vi "MoveChanGroup.vi"(7 "Up (T) / Down (F)":bool, 8 "error in (no error)":errorcluster, 9 "Rate Class":T1, 10 "ChanGroup":i32, 11 "Chassis Cfg":refnum<class "ChassisCfg.lvclass">) -> (0 "error out":errorcluster, 1 "Disregard":bool, 2 "ChanGroup Out":i32, 3 "Chassis Cfg":refnum<class "ChassisCfg.lvclass">)   [LabVIEW 2012, in "Configuration Grandmaster.lvlib" / "ChassisCfg.lvclass"]
uses:
  ChassisCfg.lvclass
  Common/Controls/TE_Designator.ctl
  ChassisCfg.lvclass/ChassisCfg.ctl
  Class Timing Group/TimingGrp.lvclass
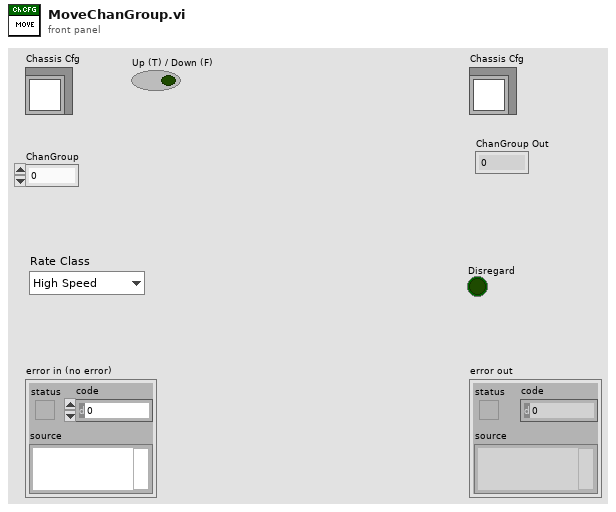
[diagram p1: front panel]
types:
  T1 = typedef "TE_Designator.ctl" = enum16{"High Speed", "Low Speed"}
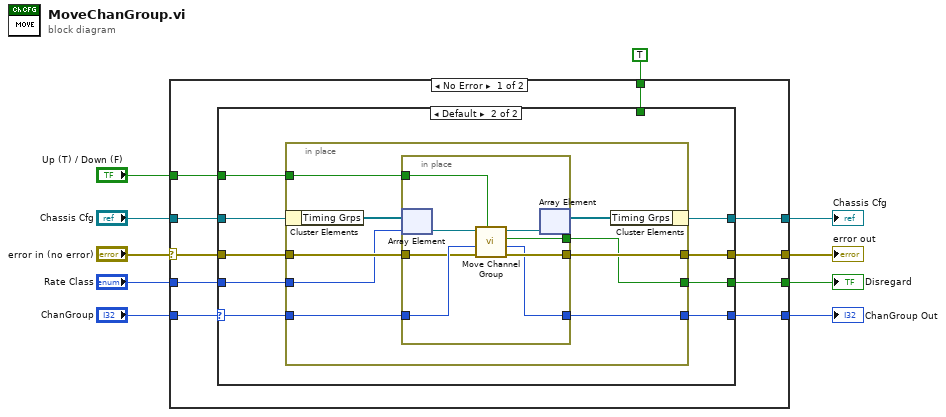
[diagram p0: block diagram]
diagram:
  n1 = case shown="No Error" "error in (no error)" {
    selector: "error in (no error)" -> [w19 w54]
    tunnel: [w17 w54] -> w9
    tunnel: [w18 w53] -> w7
    tunnel: "Chassis Cfg" -> [w20 w53]
    tunnel: "Rate Class" -> [w16 _]
    tunnel: "ChanGroup" -> [w11 w52]
    tunnel: [w15 w52] -> w4
    tunnel: [w14 w51] -> w3
    tunnel: TRUE -> [w12 w51]
    tunnel: "Up (T) / Down (F)" -> [w13 _]
    frame No Error {
      n2 = case shown="Default" w11 {
        selector: w11 -> [w23 w25]
        tunnel: w20 -> [w21 w33]
        tunnel: w19 -> [w22 w32]
        tunnel: [w21 w31] -> w18
        tunnel: [w22 w30] -> w17
        tunnel: w16 -> [_ w29]
        tunnel: [w23 w28] -> w15
        tunnel: [w24 w27] -> w14
        tunnel: w13 -> [_ w26]
        tunnel: w12 -> [w24 _]
        frame -1 {
        }
        frame Default {
          n3 = in-place {
            in-place-border: w32 -> [w40]
            in-place-border: [w39] -> w30
            in-place-border: w29 -> [w38]
            in-place-border: w25 -> [w36]
            in-place-border: [w37] -> w28
            in-place-border: [w35] -> w27
            in-place-border: w26 -> [w34]
            n4 = in-place-cluster #1(w33) -> ("Timing Grps"=w42:refnum<class "TimingGrp.lvclass">[])
            n5 = in-place {
              in-place-border: w36 -> [w50]
              in-place-border: w40 -> [w49]
              in-place-border: [w48] -> w39
              in-place-border: [w47] -> w37
              in-place-border: [w44] -> w35
              in-place-border: w34 -> [w43]
              n6 = in-place-array #2(w42, w38) -> (w46:refnum<class "TimingGrp.lvclass">)
              n7 = call "Move Channel Group.vi"("Up (T) / Down (F)"=w43, "error in (no error)"=w49, "ChanGroup"=w50, "TimingGrp in"=w46) -> ("error out"=w48:errorcluster, "ChanGroup Out"=w47:i32, "Canceled?"=w44:bool, "TimingGrp Out"=w45:refnum<class "TimingGrp.lvclass">)  [unwired: 4 in]
              n8 = in-place-array #2(w45) -> (w41:refnum<class "TimingGrp.lvclass">[])  [unwired: 1 out]
            }
            n9 = in-place-cluster #1("Timing Grps"=w41) -> (w31:refnum<class "ChassisCfg.lvclass">)
          }
        }
      }
    }
    frame Error {
    }
  }
  "error out" <- w9
  "Chassis Cfg" <- w7
  "ChanGroup Out" <- w4
  "Disregard" <- w3
